vi "Write address.vi"(8 "error in (no error)":errorcluster, 10 "address":string="localhost", 11 "Connection.TCP":refnum<class "Connection.Collection.lvclass">) -> (0 "error out":errorcluster, 3 "Connection.TCP":refnum<class "Connection.Collection.lvclass">)   [LabVIEW 2013]
uses:
  Connection.Collection.lvclass
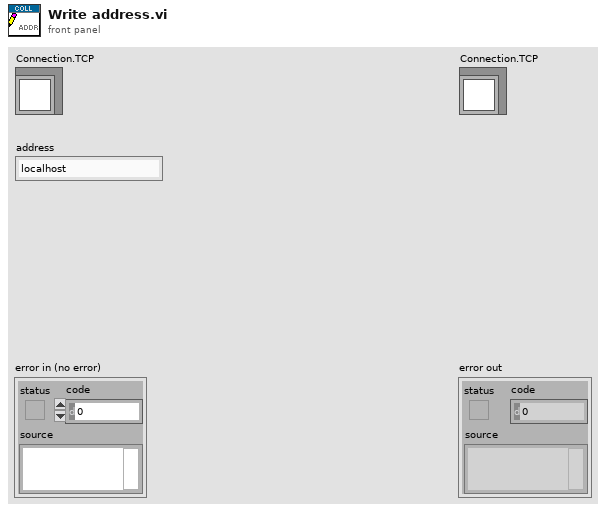
[diagram p1: front panel]
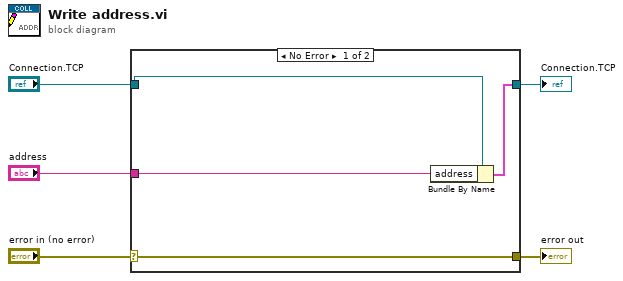
[diagram p0: block diagram]
diagram:
  n1 = case shown="No Error" "error in (no error)" {
    selector: "error in (no error)" -> [w9 w10]
    tunnel: [w9 w10] -> w4
    tunnel: [w7 w11] -> w2
    tunnel: "Connection.TCP" -> [w8 w11]
    tunnel: "address" -> [w6 _]
    frame No Error {
      n2 = Bundle By Name(cluster=w8, "address"=w6) -> (w7:cluster{})
    }
    frame Error {
    }
  }
  "error out" <- w4
  "Connection.TCP" <- w2
